vi "Logging_TDMSPath.vi"(11 "Task File Name":string) -> (3 "appended path":path)   [LabVIEW 2020]
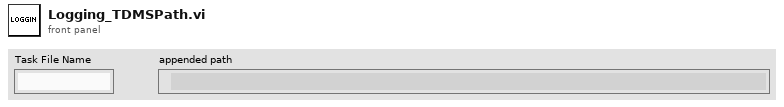
[diagram p1: front panel]
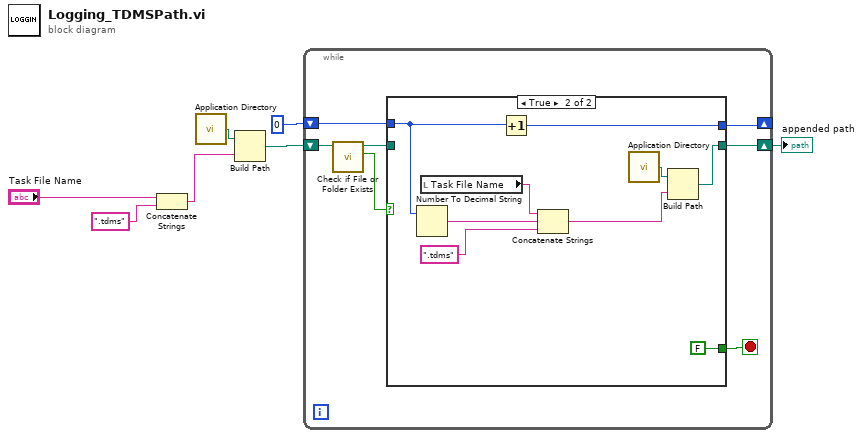
[diagram p0: block diagram]
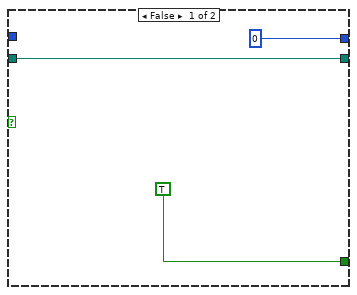
[diagram p2: hidden frame]
diagram:
  n1 = Concatenate Strings("Task File Name", ".tdms" ("string")) -> (w5:string)
  n2 = call <vilib>:"Application Directory.vi"() -> ("Application Directory"=w6:path)
  n3 = Build Path(base path=w6, name or relative path=w5) -> (appended path=w2:path)
  n4 = while {
    shift-right: [w12] -> _
    shift-left: 0 -> [w13]
    shift-right: [w11] -> w1
    shift-left: w2 -> [w10]
    stop <- w14 stop-if-true
    n5 = call <vilib>:"Check if File or Folder Exists.vi"("path"=w10) -> ("file or folder exists?"=w8:bool, "dup path"=w9:path)  [unwired: 8 in, 1 out]
    n6 = case shown="True" w8 {
      tunnel: [TRUE FALSE] -> w14
      tunnel: w13 -> [_ w20]
      tunnel: [0 w25] -> w12
      tunnel: w9 -> [w15 _]
      tunnel: [w15 w23] -> w11
      frame False {
      }
      frame True {
        n7 = Number To Decimal String(number=w20) -> (decimal integer string=w19:string)  [unwired: 1 in]
        n8 = local read "Task File Name"() -> (w22:string)
        n9 = Increment(x=w20) -> (x+1=w25:i32)
        n10 = Concatenate Strings(w22, w19, ".tdms" ("input 3")) -> (w18:string)
        n11 = call <vilib>:"Application Directory.vi"() -> ("Application Directory"=w24:path)
        n12 = Build Path(base path=w24, name or relative path=w18) -> (appended path=w23:path)
      }
    }
  }
  "appended path" <- w1
